vi "PA_Set.vi"(8 "error in (no error)":errorcluster, 9 "Target Position":i32, 10 "Axis Number":i32, 11 "Agilis in":T1) -> (0 "error out":errorcluster, 3 "Agilis out":T1)   [LabVIEW 2016, in "Drivers.lvlib" / "Agilis.lvlib"]
doc: "Starts a process to move to an absolute position. During the execution of this command, the USB communication is interrupted. After completion, the communication will resume. The execution of this command can last up to 2 minutes.\n\nMA only functions properly with devices that afeature a limit switch like models AG-LS25,AG-M050L and AG-M100L."
uses:
  Agilis.lvlib
  AgilisCmdLib Refnum.ctl
  D:/Trace Grabber/Drivers/Agilis/AgilisCmdLib.dll
  AgilisCmdLib.dll
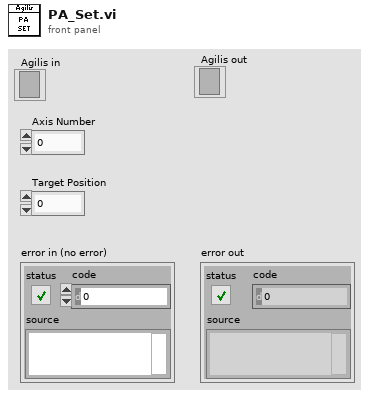
[diagram p1: front panel]
types:
  T1 = typedef "Drivers.lvlib/Agilis.lvlib/AgilisCmdLib Refnum.ctl" = refnum<k24>
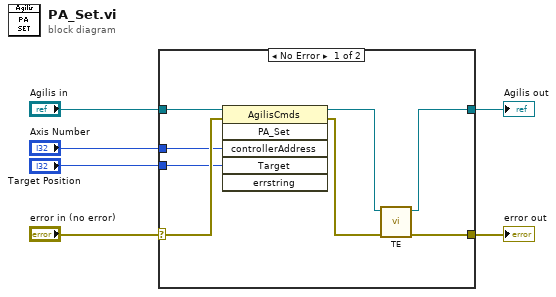
[diagram p0: block diagram]
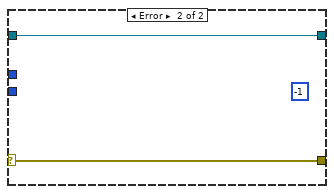
[diagram p2: hidden frame]
diagram:
  n1 = case shown="No Error" "error in (no error)" {
    selector: "error in (no error)" -> [w13 w16]
    tunnel: "Agilis in" -> [w14 w15]
    tunnel: [w7 w15] -> w4
    tunnel: [w9 w16] -> w3
    tunnel: "Axis Number" -> [w12 _]
    tunnel: "Target Position" -> [w11 _]
    frame No Error {
      n2 = invoke class="AgilisCmds" method="PA_Set"(reference=w14, error in=w13, "controllerAddress"=w12, "Target"=w11) -> (reference out=w8:T1, error out=w10:errorcluster)  [unwired: 2 in, 4 out]
      n3 = call "TE.vi"("error in (no error)"=w10, "Agilis in"=w8) -> ("error out"=w9:errorcluster, "Agilis out"=w7:T1)  [unwired: 8 in]
    }
    frame Error {
      (unwired) -1 ("Target")
    }
  }
  "Agilis out" <- w4
  "error out" <- w3
